vi "RequestTargetInfo.vi"() -> (1 "haveInfo":bool, 3 "Location":T1)   [LabVIEW 2012]
uses:
  TargetData.ctl
  Vision Global Data.vi
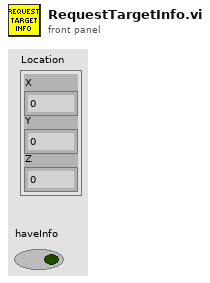
[diagram p1: front panel]
types:
  T1 = typedef "TargetData.ctl" = cluster{"X":dbl, "Y":dbl, "Z":dbl}
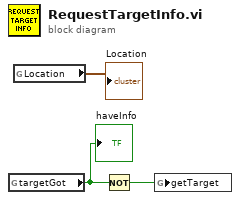
[diagram p0: block diagram]
diagram:
  n1 = global read "Vision Global Data.vi" "targetGot"() -> (w3:bool)
  "haveInfo" <- w3
  n2 = global read "Vision Global Data.vi" "Location"() -> (→"Location":T1)
  n3 = Not(x=w3) -> (.not. x?=w2:bool)
  n4 = global write "Vision Global Data.vi" "getTarget"(w2) -> ()
